vi "Get-value-reference.vi"(8 "error in (no error)":errorcluster, 11 "Correct params in":refnum<class "CV-Correction.lvclass">) -> (0 "error out":errorcluster, 3 "Correct. params. ref.":refnum<data-value>)   [LabVIEW 2013, in "CameraVision.lvlib" / "CV-Correction.lvclass"]
uses:
  CV-Correction.lvclass
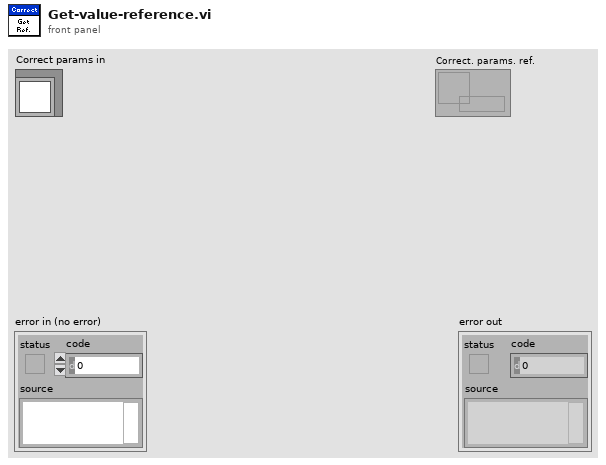
[diagram p1: front panel]
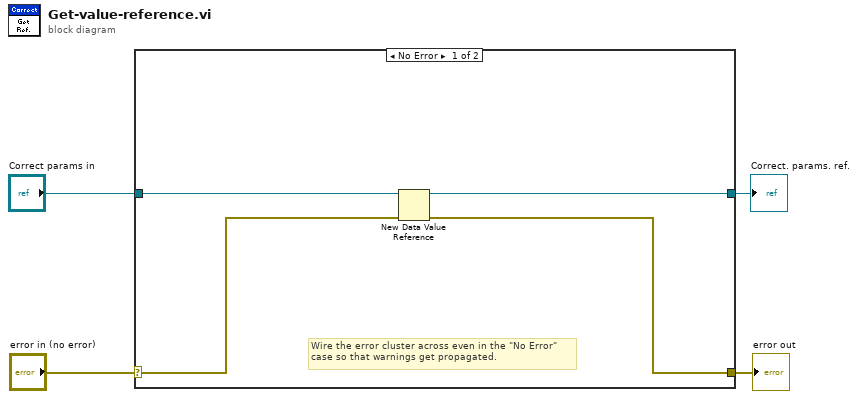
[diagram p0: block diagram]
diagram:
  n1 = case shown="No Error" "error in (no error)" {
    selector: "error in (no error)" -> [w6 w9]
    tunnel: [w5 w9] -> w3
    tunnel: "Correct params in" -> [w8 _]
    tunnel: [w7 _] -> w1
    frame No Error {
      # "Wire the error cluster across even in the \"No Error\"\ncase so that warnings get propagated."
      n2 = New Data Value Reference(data value=w8, error in=w6) -> (data value reference=w7:refnum<data-value>, error out=w5:errorcluster)
    }
    frame Error {
    }
  }
  "error out" <- w3
  "Correct. params. ref." <- w1
